vi "serialZap_p.vi"(2 "serialBoard":u16(ring) items=["DEVIL", "M17"], 3 "subID2 (0)":u32, 4 "subID1 (0)":u32 format="%.0x", 5 "baseAdderess":u32=3774873600 format="%.0x") -> (0 "errorSpec":i32, 1 "errorCode":cdb format="%.2f")   [LabVIEW 2010]
doc: "cleans the content of the input buffer of the serial port indicated by \"subID1\" and \"subID2\".\nWARNING: remember to setup the serial channel before running this routine using:\n1. \"serialInitialize.vi\" for hardware setup;\n2. \"serialConfigure\" for software setup."
uses:
  <userlib>/libcommon_serial/libcommon_serial.lvlib
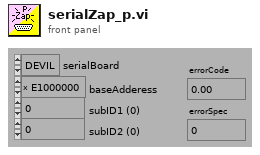
[diagram p1: front panel]
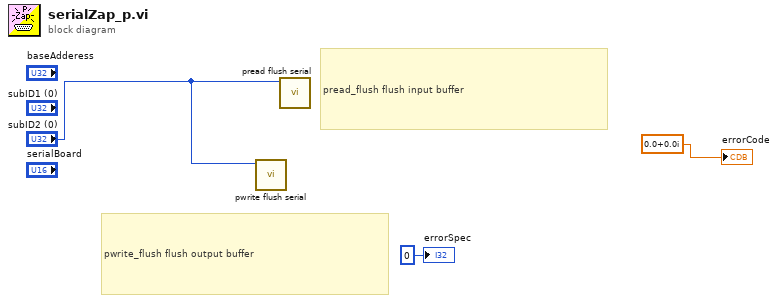
[diagram p0: block diagram]
diagram:
  # "pwrite_flush flush output buffer"
  # "pread_flush flush input buffer"
  n1 = call <userlib>:"pwrite flush serial.vi"("resourceId"="subID2 (0)") -> ()  [unwired: 10 in, 1 out]
  n2 = call <userlib>:"pread flush serial.vi"("resourceId"="subID2 (0)") -> ()  [unwired: 10 in, 1 out]
  "errorCode" <- cdb 0.0+0.0i ("errorCode")
  "errorSpec" <- 0 ("errorSpec")
